vi "Save Transport DAT File.vi"(8 "error in (no error)":errorcluster, 10 "Data (Row)":dbl[](array[numeric]), 11 "Control Experiment in":refnum<class "AFM Control.lvclass">) -> (0 "error out":errorcluster, 3 "Control Experiment out":refnum<class "AFM Control.lvclass">)   [LabVIEW 2016]
uses:
  <userlib>/LevyLab/LV to ITX/LVtoITX.lvclass
  <userlib>/LevyLab/LV to ITX/Main/LV to DAT 1D.vi
  AFM Control.lvclass
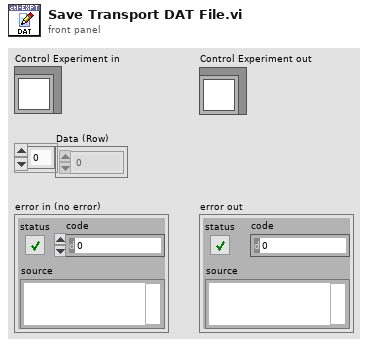
[diagram p1: front panel]
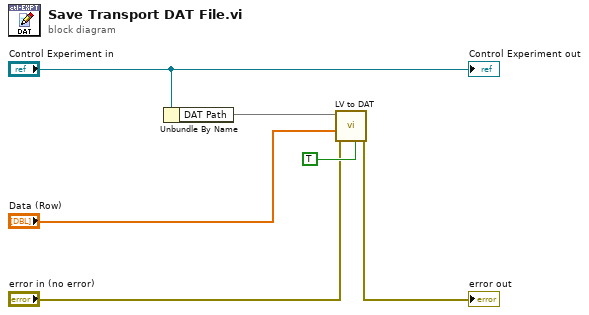
[diagram p0: block diagram]
diagram:
  n1 = Unbundle By Name("Control Experiment in") -> ("DAT Path"=w3)
  n2 = call-poly <userlib>:"LV to DAT.vi"("append to file? (new file:F)"=TRUE, "error in"="error in (no error)", "Data"="Data (Row)", "path"=w3) -> ("error out"=→"error out":errorcluster)  [unwired: 6 in, 1 out]
  "Control Experiment out" <- "Control Experiment in"
